vi "GenTargetAngles.vi"() -> ()   [LabVIEW 2016]
uses:
  Classes/CAlex2/TypeDef/CAlexVersion.ctl
  Sim&Process/DataProcess/CAlex2-Data/CAlex2_Data.lvclass
  C:/Users/randh/Desktop/BILATERAL/CAlex2-controller/Sim&Process/DataProcess/ExpData/ExpData.lvclass
  Sim&Process/DataProcess/CAlex2-Data/PropertyNodes/Get_JointAngles.vi
  <vilib>/Utility/file.llb/Write Delimited Spreadsheet (string).vi
  <vilib>/Utility/file.llb/Write Delimited Spreadsheet (DBL).vi
  Sim&Process/DataProcess/ExpData/ExpData.lvclass
  <vilib>/AuZn/auzn custom VIs/AuZnCustomVI.lvlib
  Classes/CAlex2/CAlex2.lvclass
panel:
  out "Xmin":dbl
  out "Xmax":dbl
  out "Ymin":dbl
  out "Ymax":dbl
  out "CAlexVersion":T1
  out "AveragedJointAngle":dbl[][](array[numeric])
  out "TargetJointAngle":dbl[][](array[numeric])
  out "TargetTraj":dbl[][](array[numeric])
  in  "Save":bool
  in  "ScalingCoef Knee":dbl=1.0 format="%#_13g"
  out "Leg Length":cluster{"Thigh":dbl, "Shank":dbl}
  in  "Scale Method":T2(ring)
  in  "OutputLength":i32=500
  in  "ScalingCoef Hip":dbl=1.3 format="%#_13g"
  out "Array":dbl[](array[numeric])
  in  "Update":bool
  in  "Open":bool
  in  "stop":bool
  in  "EndTime":dbl=240.0
  in  "StartTime":dbl=60.0
  in  "Cut":bool
  out "AveragedTrajectory":dbl[][](graph)
  out "Averaged":cluster{"Mean":dbl[], "Mean":dbl[]}[](graph)
  out "Stacked":T3(graph)
  out "Ankle - X":dbl[][](graph)
  in  "Cut Parameter":dbl=100.0
  in  "Path":path=path "C:/Users/Rand/Desktop/s09_fw_lap1 (1).txt"
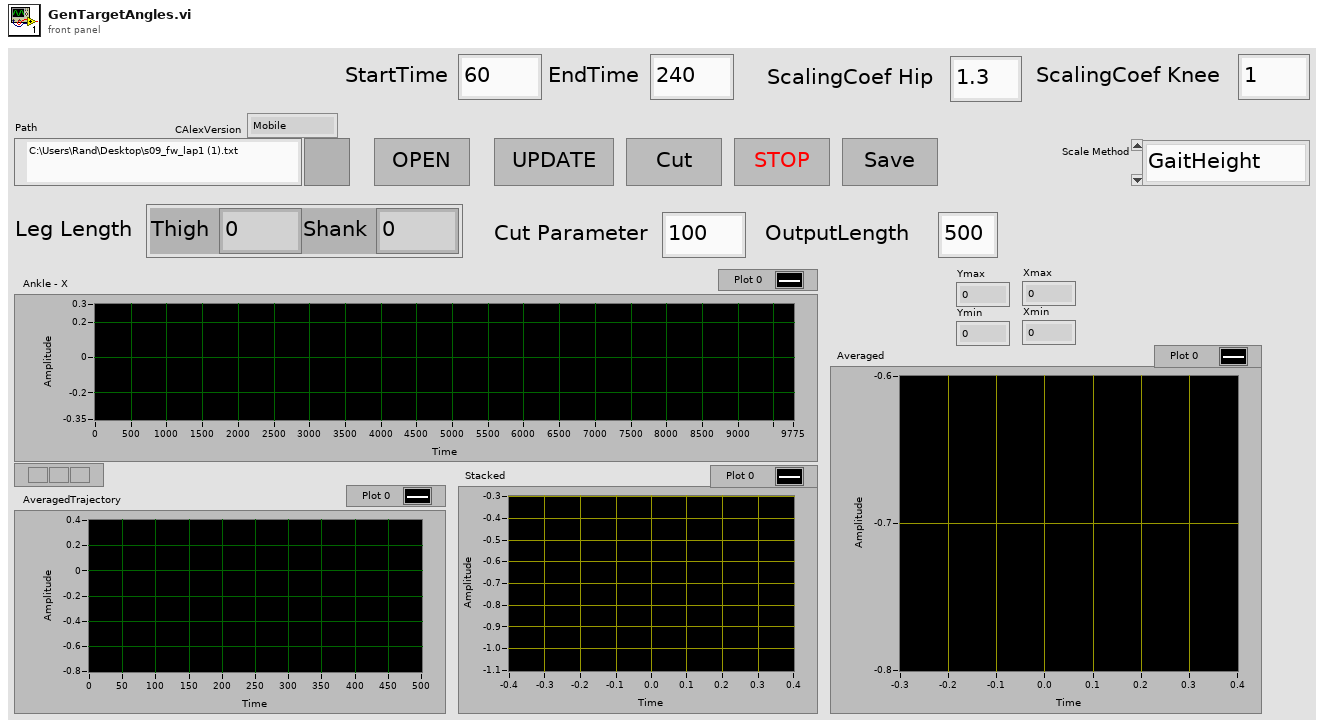
[diagram p1: front panel]
types:
  T1 = typedef "CAlex2.lvclass/CAlexVersion.ctl" = enum16{"Mobile", "Squat", "Soft", "Treadmill"}
  T2 = enum16{"GaitHeight", "Angle", "Step Length Anterior", "Step Length Posterior", "Posterior Length & Height", "Anterior Length & Height"}
  T3 = cluster{"DataAccess:WaistPosition":dbl[], "DataAccess:WaistPosition":dbl[]}
  T4 = enum16{"open", "replace", "create", "open or create", "replace or create", "replace or create with confirmation"}
  T5 = cluster{"ThighLt":dbl, "ShankLt":dbl, "HipWd":dbl}
  T6 = cluster{"ScaledGait":dbl[], "ScaledGait":dbl[]}[]
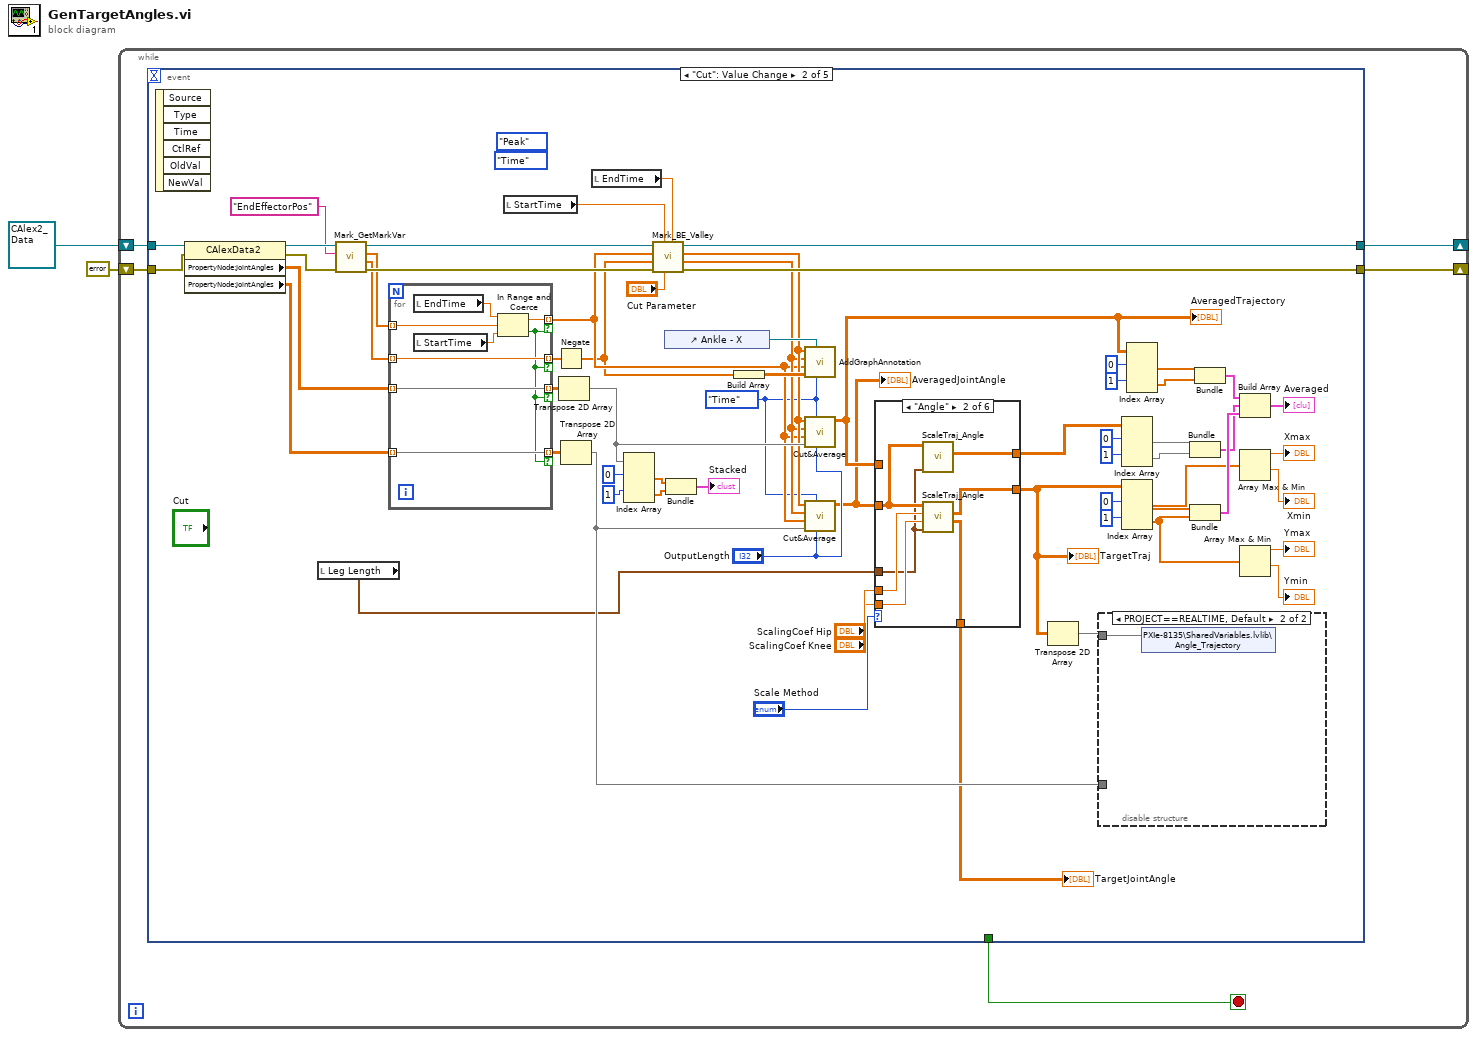
[diagram p0: block diagram]
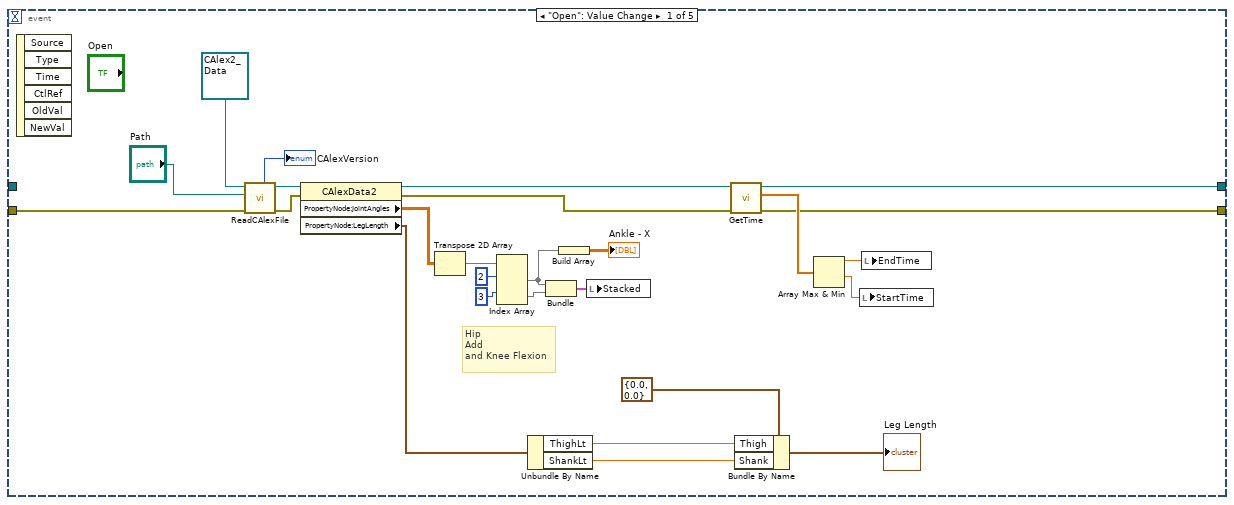
[diagram p2: hidden frame]
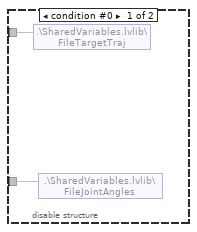
[diagram p3: hidden frame]
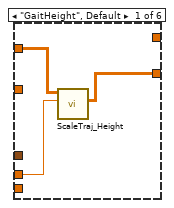
[diagram p4: hidden frame]
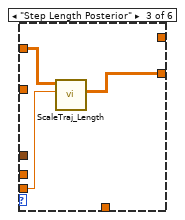
[diagram p5: hidden frame]
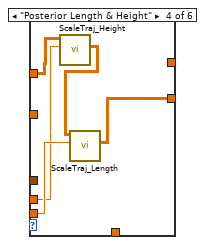
[diagram p6: hidden frame]
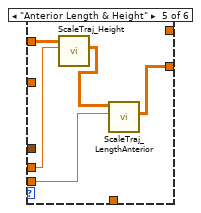
[diagram p7: hidden frame]
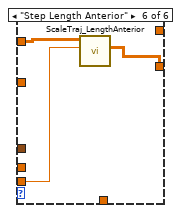
[diagram p8: hidden frame]
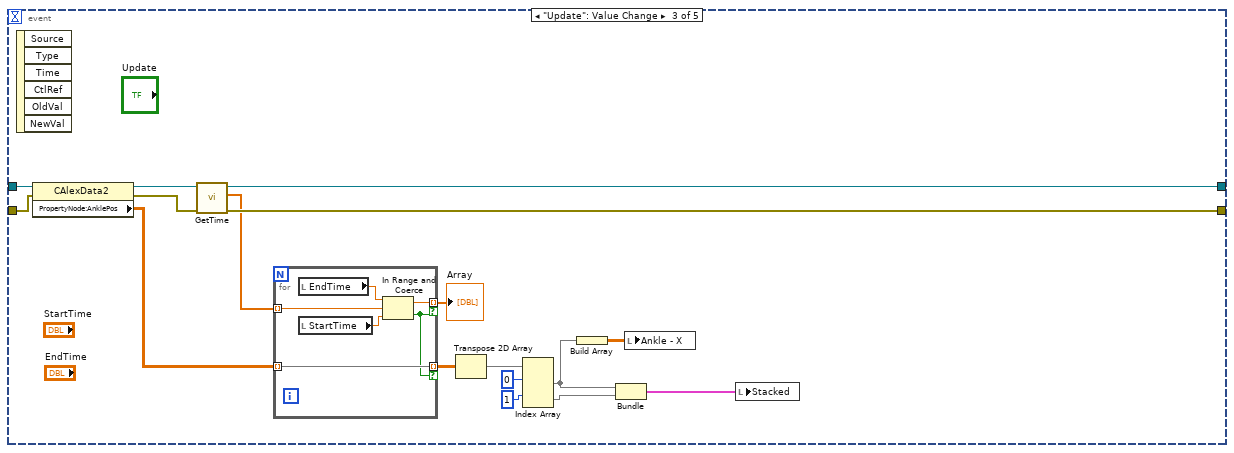
[diagram p9: hidden frame]
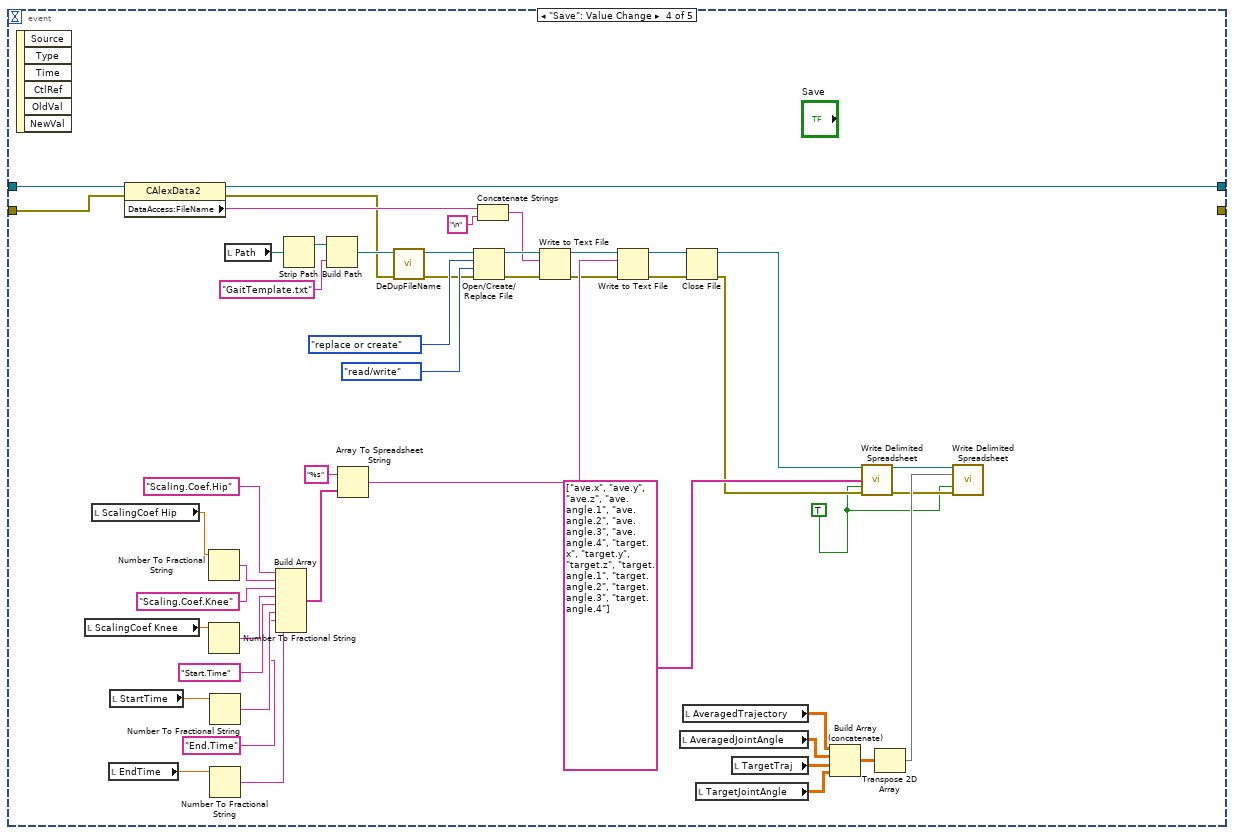
[diagram p10: hidden frame]
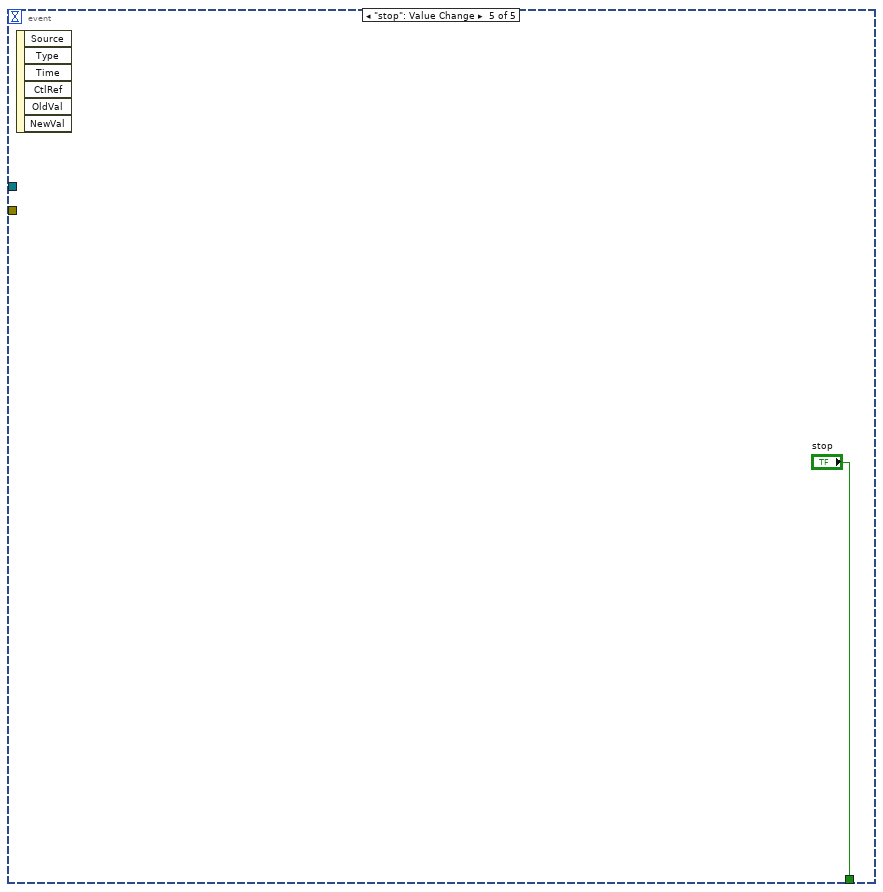
[diagram p11: hidden frame]
diagram:
  n1 = while {
    shift-right: [w4] -> _
    shift-left: refnum<class "CAlex2_Data.lvclass"> refnum ("CAlexData") -> [w7]
    shift-right: [w5] -> _
    shift-left: errorcluster {"status"=FALSE, "code"=0, "source"=""} ("error out") -> [w6]
    stop <- w3 stop-if-true
    n2 = event shown="[1] \"Cut\": Value Change" {
      selector: _ -> [_ _ _ _ _]
      dyn-events: _ -> [_ _ _ _ _]
      timeout: _ -> [_ _ _ _ _]
      tunnel: w7 -> [_ w89 w148 w170 _]
      tunnel: w6 -> [w23 w87 w147 w171 _]
      tunnel: [w20 w79 w139 _ _] -> w5
      tunnel: [w22 w78 w141 w169 _] -> w4
      tunnel: [_ _ _ _ "stop"] -> w3
      event "Open": Value Change {
        # "Hip\nAdd\nand Knee Flexion"
        n3 = event-data() -> ()  [unwired: 1 in, 6 out]
        n4 = call "ReadCAlexFile.vi"("error in (no error)"=w23, "ExpData File Path"="Path", "CAlexData2"=refnum<class "CAlex2_Data.lvclass"> refnum ("CAlexData")) -> ("error out"=w17:errorcluster, "CAlexData 2"=w19:refnum<class "CAlex2_Data.lvclass">, "CAlexVersion"=→"CAlexVersion":T1)  [unwired: 6 in]
        n5 = property class="CAlexData2"(reference=w19, error in=w17) -> (reference out=w18:refnum<class "CAlex2_Data.lvclass">, error out=w16:errorcluster, "PropertyNode:JointAngles"=w15:dbl[][], "PropertyNode:LegLength"=w14:T5)
        n6 = Transpose 2D Array(2D array=w15) -> (transposed array=w9:dbl[][])
        n7 = Index Array(array=w9, index (row) #1=2 ("index (row)"), index (row) #2=3 ("index (row)")) -> (element #1=w27:dbl[], element #2=w26:dbl[])  [unwired: 2 in]
        n8 = Unbundle By Name(w14) -> ("ThighLt"=w12:dbl, "ShankLt"=w11:dbl)
        n9 = Bundle(w27, w26) -> (w29:cluster{dbl[], dbl[]})  [unwired: 1 in]
        n10 = Build Array(w27) -> (→"Ankle - X":dbl[][])
        n11 = local write "Stacked"(w29) -> ()
        n12 = call "GetTime.vi"("error in (no error)"=w16, "ExpData in"=w18) -> ("error out"=w20:errorcluster, "Time"=w21:dbl[], "ExpData out"=w22:refnum<class "CAlex2_Data.lvclass">)  [unwired: 7 in]
        n13 = Bundle By Name(cluster=cluster{"Thigh":dbl, "Shank":dbl} {"Thigh"=0.0, "Shank"=0.0} ("Leg Length"), "Thigh"=w12, "Shank"=w11) -> (→"Leg Length":cluster{"Thigh":dbl, "Shank":dbl})
        n14 = Array Max & Min(array=w21) -> (max value=w33:dbl, min value=w32:dbl)  [unwired: 2 out]
        n15 = local write "StartTime"(w32) -> ()
        n16 = local write "EndTime"(w33) -> ()
      }
      event "Cut": Value Change {
        w72 = enum16{"Time", "Percentage", "Index"}."Time" ("Input Type")
        (unwired) enum16{"Peak", "Valley"}."Peak" ("Peak/Valley")
        (unwired) enum16{"Time", "Percentage", "Index"}."Time" ("Output Type")
        n17 = event-data() -> ()  [unwired: 1 in, 6 out]
        n18 = property class="CAlexData2"(reference=w89, error in=w87) -> (reference out=w88:refnum<class "CAlex2_Data.lvclass">, error out=w86:errorcluster, "PropertyNode:JointAngles"=w45:dbl[][], "PropertyNode:JointAngles"=w44:dbl[][])
        n19 = local read "Leg Length"() -> (w47:cluster{"Thigh":dbl, "Shank":dbl})
        n20 = call "Mark_GetMarkVar.vi"("error in (no error)"=w86, "VarName"="EndEffectorPos", "ExpData in"=w88) -> ("error out"=w96:errorcluster, "MarkVar"=w94:dbl[], "Time"=w95:dbl[], "ExpData out"=w90:refnum<class "CAlex2_Data.lvclass">)  [unwired: 3 in, 2 out]
        n21 = for {
          tunnel: w95 -> [w134] mode=indexing
          tunnel: w94 -> [w130] mode=indexing
          tunnel: [w131] -> w74 mode=indexing if=w127
          tunnel: [w130] -> w93 mode=indexing if=w127
          tunnel: w45 -> [w129] mode=indexing
          tunnel: [w129] -> w85 mode=indexing if=w127
          tunnel: w44 -> [w128] mode=indexing
          tunnel: [w128] -> w69 mode=indexing if=w127
          n22 = local read "EndTime"() -> (w132:dbl)
          n23 = local read "StartTime"() -> (w133:dbl)
          n24 = In Range and Coerce(upper limit=w132, x=w134, lower limit=w133) -> (coerced(x)=w131:dbl, In Range?=w127:bool)
        }
        n25 = local read "StartTime"() -> (w42:dbl)
        n26 = Negate(x=w93) -> (-x=w41:dbl[])
        n27 = Transpose 2D Array(2D array=w85) -> (transposed array=w77:dbl[][])
        n28 = Transpose 2D Array(2D array=w69) -> (transposed array=w57:dbl[][])
        n29 = local read "EndTime"() -> (w43:dbl)
        n30 = Index Array(array=w77, index (row) #1=0 ("index (row)"), index (row) #2=1 ("index (row)")) -> (element #1=w82:dbl[], element #2=w81:dbl[])  [unwired: 2 in]
        n31 = call "Mark_BE_Valley.vi"("End Time"=w43, "HalfWidth"="Cut Parameter", "Start Time"=w42, "error in (no error)"=w96, "Input"=w41, "Time"=w74, "CarexData In"=w90) -> ("error out"=w79:errorcluster, "End"=w75:dbl[], "Begin"=w76:dbl[], "CarexData Out"=w78:refnum<class "CAlex2_Data.lvclass">)  [unwired: 1 in]
        n32 = control-ref of="Ankle - X"() -> (w91:refnum<vi>)
        n33 = Bundle(w82, w81) -> (→"Stacked":cluster{dbl[], dbl[]})  [unwired: 1 in]
        n34 = Build Array(w41) -> (w92:dbl[][])
        n35 = call <vilib>:"AddGraphAnnotation.vi"("Input Type (Time)"=w72, "WaveformGraph in"=w91, "Array"=w92, "Time"=w74, "Valleys  (Yellow)"=w75, "Peaks (Red)"=w76) -> ()  [unwired: 4 in, 2 out]
        n36 = call <vilib>:"Cut&Average.vi"("Dilate Length (200)"="OutputLength", "Input Type (Time)"=w72, "Data"=w77, "Time"=w74, "End"=w75, "Begin"=w76) -> ("Mean"=w60:dbl[][])  [unwired: 5 out]
        "AveragedTrajectory" <- w60
        n37 = call <vilib>:"Cut&Average.vi"("Dilate Length (200)"="OutputLength", "Input Type (Time)"=w72, "Data"=w57, "Time"=w74, "End"=w75, "Begin"=w76) -> ("Mean"=w56:dbl[][])  [unwired: 5 out]
        "AveragedJointAngle" <- w56
        n38 = case shown="\"Angle\"" "Scale Method" {
          tunnel: [w102 w109 w111 w116 w119 w124] -> w58
          tunnel: w56 -> [_ w106 _ _ _ _]
          tunnel: w47 -> [_ w105 _ _ _ _]
          tunnel: "ScalingCoef Hip" -> [w103 w110 _ w117 w121 _]
          tunnel: w60 -> [w101 _ w112 w115 w122 w126]
          tunnel: "ScalingCoef Knee" -> [_ w108 w113 w118 w120 w125]
          tunnel: [_ w107 _ _ _ _] -> w55
          tunnel: [_ w104 _ _ _ _] -> w50
          frame "GaitHeight", Default {
            n39 = call "ScaleTraj_Height.vi"("ScalingCoef"=w103, "Averaged Gait"=w101) -> ("ScaledGait"=w102:dbl[][])  [unwired: 8 in, 1 out]
          }
          frame "Angle" {
            n40 = call "ScaleTraj_Angle.vi"("ArmLength"=w105, "AverageJointAngles"=w106) -> ("ScaledGait"=w104:dbl[][])  [unwired: 8 in, 1 out]
            n41 = call "ScaleTraj_Angle.vi"("ArmLength"=w105, "ScalingCoef Knee (1)"=w108, "ScalingCoef Hip (1)"=w110, "AverageJointAngles"=w106) -> ("ScaledJointAngles"=w107:dbl[][], "ScaledGait"=w109:dbl[][])  [unwired: 6 in]
          }
          frame "Step Length Posterior" {
            n42 = call "ScaleTraj_Length.vi"("ScalingCoef"=w113, "Averaged Gait"=w112) -> ("ScaledGait"=w111:dbl[][])  [unwired: 8 in, 1 out]
          }
          frame "Posterior Length & Height" {
            n43 = call "ScaleTraj_Height.vi"("ScalingCoef"=w117, "Averaged Gait"=w115) -> ("ScaledGait"=w114:dbl[][])  [unwired: 8 in, 1 out]
            n44 = call "ScaleTraj_Length.vi"("ScalingCoef"=w118, "Averaged Gait"=w114) -> ("ScaledGait"=w116:dbl[][])  [unwired: 8 in, 1 out]
          }
          frame "Anterior Length & Height" {
            n45 = call "ScaleTraj_Height.vi"("ScalingCoef"=w121, "Averaged Gait"=w122) -> ("ScaledGait"=w123:dbl[][])  [unwired: 8 in, 1 out]
            n46 = call "ScaleTraj_LengthAnterior.vi"("ScalingCoef"=w120, "Averaged Gait"=w123) -> ("ScaledGait"=w119:dbl[][])  [unwired: 8 in, 1 out]
          }
          frame "Step Length Anterior" {
            n47 = call "ScaleTraj_LengthAnterior.vi"("ScalingCoef"=w125, "Averaged Gait"=w126) -> ("ScaledGait"=w124:dbl[][])  [unwired: 8 in, 1 out]
          }
        }
        "TargetTraj" <- w58
        "TargetJointAngle" <- w55
        n48 = Transpose 2D Array(2D array=w58) -> (transposed array=w40:dbl[][])
        n49 = disable-structure shown="PROJECT==REALTIME, Default" {
          disable-tunnel: w40 -> [w99 w100]
          disable-tunnel: w57 -> [w98 _]
          frame condition #0 {
            n50 = shared-variable ".\\SharedVariables.lvlib\\FileTargetTraj"(w99) -> ()  [unwired: 1 in, 1 out]
            n51 = shared-variable ".\\SharedVariables.lvlib\\FileJointAngles"(w98) -> ()  [unwired: 1 in, 1 out]
          }
          frame condition #1 (active) {
            n52 = shared-variable "PXIe-8135\\SharedVariables.lvlib\\Angle_Trajectory"(w100) -> ()  [unwired: 1 in, 1 out]
          }
        }
        n53 = Index Array(array=w50, index (row) #1=0 ("index (row)"), index (row) #2=1 ("index (row)")) -> (element #1=w52:dbl[], element #2=w51:dbl[])  [unwired: 2 in]
        n54 = Index Array(array=w58, index (row) #1=0 ("index (row)"), index (row) #2=1 ("index (row)")) -> (element #1=w36:dbl[], element #2=w39:dbl[])  [unwired: 2 in]
        n55 = Index Array(array=w60, index (row) #1=0 ("index (row)"), index (row) #2=1 ("index (row)")) -> (element #1=w65:dbl[], element #2=w66:dbl[])  [unwired: 2 in]
        n56 = Bundle("ScaledGait"=w52, "ScaledGait"=w51) -> (w48:cluster{"ScaledGait":dbl[], "ScaledGait":dbl[]})  [unwired: 1 in]
        n57 = Bundle("ScaledGait"=w36, "ScaledGait"=w39) -> (w62:cluster{"ScaledGait":dbl[], "ScaledGait":dbl[]})  [unwired: 1 in]
        n58 = Bundle("Mean"=w65, "Mean"=w66) -> (w49:cluster{"Mean":dbl[], "Mean":dbl[]})  [unwired: 1 in]
        n59 = Build Array(w49, w48, w62) -> (→"Averaged":T6)
        n60 = Array Max & Min(array=w36) -> (max value=→"Xmax":dbl, min value=→"Xmin":dbl)  [unwired: 2 out]
        n61 = Array Max & Min(array=w39) -> (max value=→"Ymax":dbl, min value=→"Ymin":dbl)  [unwired: 2 out]
      }
      event "Update": Value Change {
        n62 = event-data() -> ()  [unwired: 1 in, 6 out]
        n63 = property class="CAlexData2"(reference=w148, error in=w147) -> (reference out=w142:refnum<class "CAlex2_Data.lvclass">, error out=w140:errorcluster, "PropertyNode:AnklePos"=w137:dbl[][])
        n64 = call "GetTime.vi"("error in (no error)"=w140, "ExpData in"=w142) -> ("error out"=w139:errorcluster, "Time"=w138:dbl[], "ExpData out"=w141:refnum<class "CAlex2_Data.lvclass">)  [unwired: 7 in]
        n65 = for {
          tunnel: w138 -> [w157] mode=indexing
          tunnel: [w154] -> w146 mode=indexing if=w152
          tunnel: w137 -> [w153] mode=indexing
          tunnel: [w153] -> w136 mode=indexing if=w152
          n66 = local read "EndTime"() -> (w155:dbl)
          n67 = local read "StartTime"() -> (w156:dbl)
          n68 = In Range and Coerce(upper limit=w155, x=w157, lower limit=w156) -> (coerced(x)=w154:dbl, In Range?=w152:bool)
        }
        "Array" <- w146
        n69 = Transpose 2D Array(2D array=w136) -> (transposed array=w135:dbl[][])
        n70 = Index Array(array=w135, index (row) #1=0 ("index (row)"), index (row) #2=1 ("index (row)")) -> (element #1=w144:dbl[], element #2=w143:dbl[])  [unwired: 2 in]
        n71 = Build Array(w144) -> (w145:dbl[][])
        n72 = Bundle(w144, w143) -> (w149:cluster{dbl[], dbl[]})  [unwired: 1 in]
        n73 = local write "Ankle - X"(w145) -> ()
        n74 = local write "Stacked"(w149) -> ()
      }
      event "Save": Value Change {
        w158 = TRUE ("append to file? (new file:F)")
        n75 = event-data() -> ()  [unwired: 1 in, 6 out]
        n76 = local read "ScalingCoef Knee"() -> (w196:dbl)
        n77 = local read "ScalingCoef Hip"() -> (w197:dbl)
        n78 = local read "EndTime"() -> (w181:dbl)
        n79 = local read "StartTime"() -> (w180:dbl)
        n80 = property class="CAlexData2"(reference=w170, error in=w171) -> (reference out=w169:refnum<class "CAlex2_Data.lvclass">, error out=w159:errorcluster, "DataAccess:FileName"=w168:string)
        n81 = Number To Fractional String(number=w197) -> (F-format string=w194:string)  [unwired: 3 in]
        n82 = Number To Fractional String(number=w196) -> (F-format string=w192:string)  [unwired: 3 in]
        n83 = Number To Fractional String(number=w180) -> (F-format string=w178:string)  [unwired: 3 in]
        n84 = Number To Fractional String(number=w181) -> (F-format string=w176:string)  [unwired: 3 in]
        n85 = local read "Path"() -> (w205:path)
        n86 = Build Array("Scaling.Coef.Hip" ("name or relative path"), w194, "Scaling.Coef.Knee" ("name or relative path"), w192, "Start.Time" ("name or relative path"), w178, "End.Time" ("name or relative path"), w176) -> (w191:string[])
        n87 = Strip Path(path=w205) -> (stripped path=w203:path)  [unwired: 1 out]
        n88 = Build Path(base path=w203, name or relative path="GaitTemplate.txt") -> (appended path=w162:path)
        n89 = Array To Spreadsheet String(array=w191, 3:"%s" ("format string")) -> (spreadsheet string=w190:string)  [unwired: 1 in]
        n90 = call <vilib>:"DeDupFileName.vi"("error in (no error)"=w159, "Path"=w162) -> ("error out"=w160:errorcluster, "Out Path"=w161:path)  [unwired: 7 in, 1 out]
        n91 = Open/Create/Replace File(file path (use dialog)=w161, error in=w160, operation (0:open)=T4."replace or create", access (0:read/write)=enum16{"read/write", "read-only", "write-only"}."read/write") -> (refnum out=w175:refnum<file>, error out=w173:errorcluster)  [unwired: 2 in, 1 out]
        n92 = Concatenate Strings(w168, "\n" ("string")) -> (w167:string)
        n93 = Write to Text File(file (use dialog)=w175, text=w167, error in=w173) -> (refnum out=w174:refnum<file>, error out=w172:errorcluster)  [unwired: 1 in, 1 out]
        n94 = Write to Text File(file (use dialog)=w174, text=w190, error in=w172) -> (refnum out=w186:refnum<file>, error out=w187:errorcluster)  [unwired: 1 in, 1 out]
        n95 = local read "AveragedJointAngle"() -> (w183:dbl[][])
        n96 = local read "AveragedTrajectory"() -> (w184:dbl[][])
        n97 = Close File(refnum=w186, error in=w187) -> (path=w185:path, error out=w164:errorcluster)
        n98 = local read "TargetJointAngle"() -> (w201:dbl[][])
        n99 = local read "TargetTraj"() -> (w204:dbl[][])
        n100 = Build Array (concatenate)(w184, w183, w204, w201) -> (w200:dbl[][])
        n101 = call-poly <vilib>:"Write Delimited Spreadsheet.vi"("file path (dialog if empty)"=w185, "1D data"=string[] ["ave.x", "ave.y", "ave.z", "ave.angle.1", "ave.angle.2", "ave.angle.3", "ave.angle.4", "target.x", "target.y", "target.z", "target.angle.1", "target.angle.2", "target.angle.3", "target.angle.4"], "append to file? (new file:F)"=w158, "error in (no error)"=w164) -> ("new file path (Not A Path if cancelled)"=w199:path, "error out"=w163:errorcluster)  [unwired: 10 in]
        n102 = Transpose 2D Array(2D array=w200) -> (transposed array=w198:dbl[][])
        n103 = call-poly <vilib>:"Write Delimited Spreadsheet.vi"("file path (dialog if empty)"=w199, "2D data"=w198, "append to file? (new file:F)"=w158, "error in (no error)"=w163) -> ()  [unwired: 10 in, 2 out]
      }
      event "stop": Value Change {
        n104 = event-data() -> ()  [unwired: 1 in, 6 out]
      }
    }
  }
